vi "bob tilt from parameters.vi"(5 "y0":dbl, 6 "z0":dbl, 7 "x0":dbl, 8 "t":dbl, 9 "phi_dot":dbl, 10 "phi0":dbl, 11 "bob tilt":dbl) -> (2 "derivatives (i,j) = dOut(i) / dParam(j)":dbl[][](array[numeric]), 3 "Out = (x,y,z,tx,ty,BrV)":dbl[](array[numeric]))   [LabVIEW 2017]
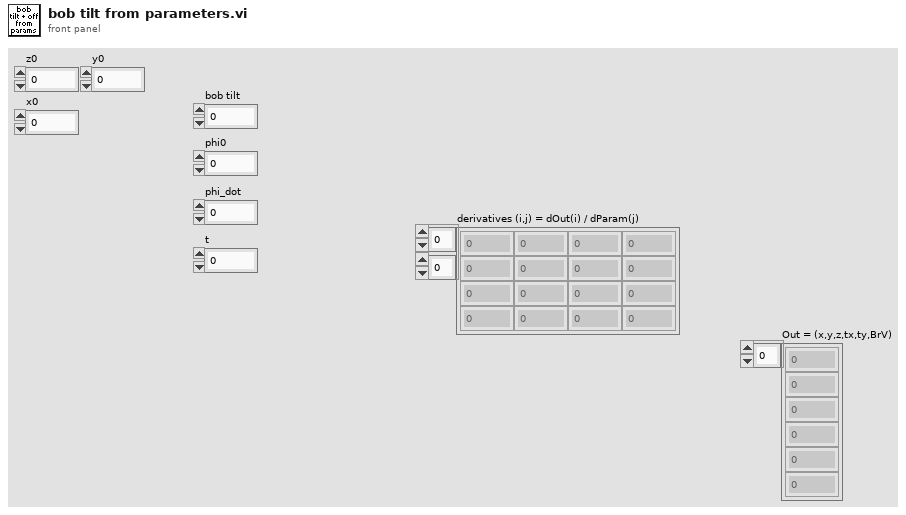
[diagram p1: front panel]
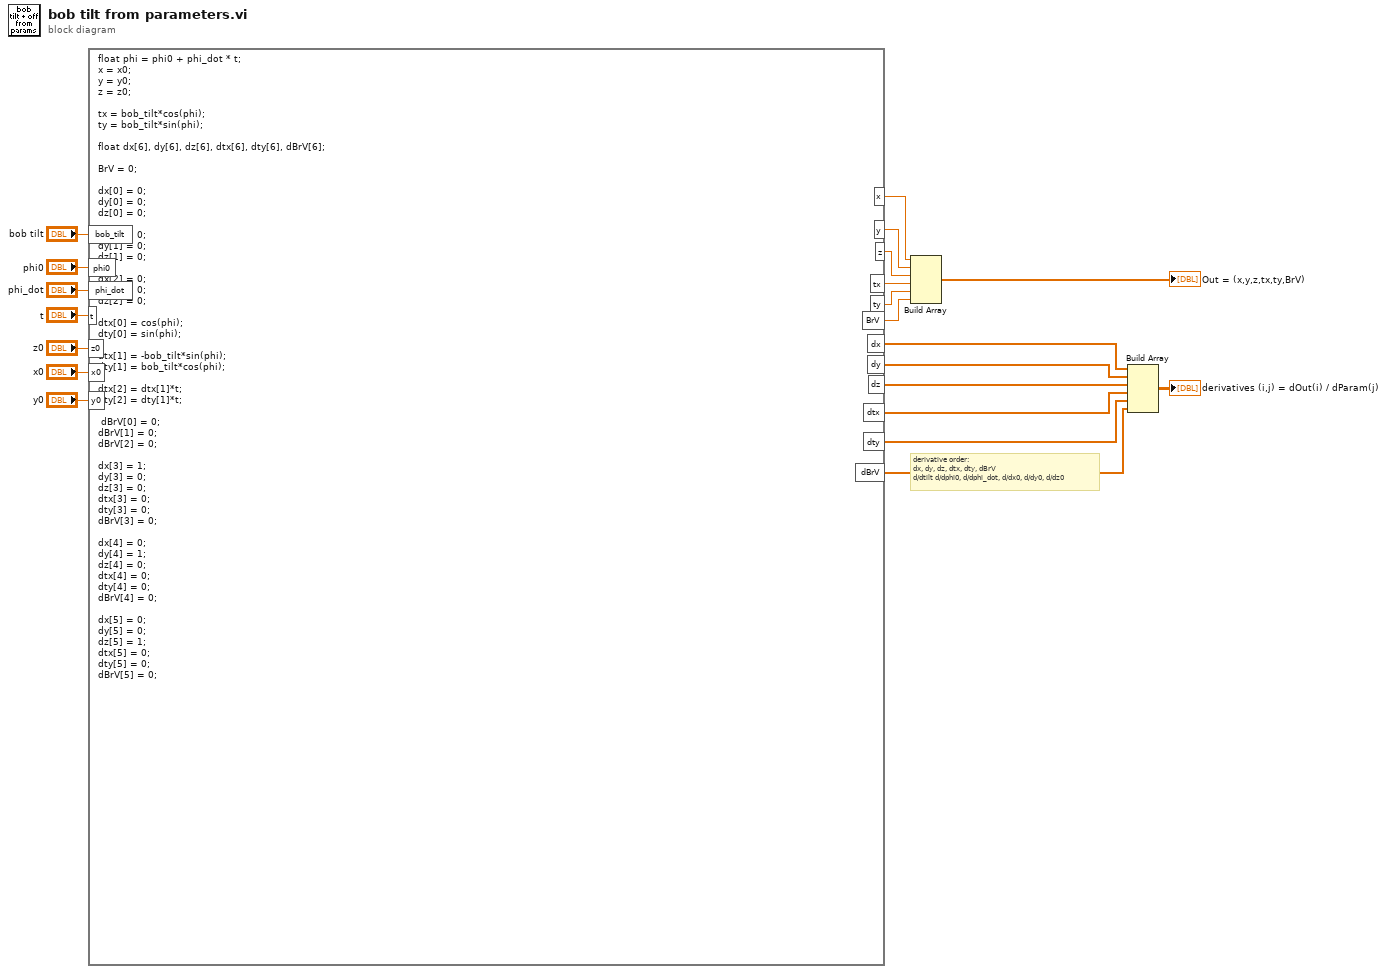
[diagram p0: block diagram]
diagram:
  # "derivative order:\ndx, dy, dz, dtx, dty, dBrV\nd/dtilt d/dphi0, d/dphi_dot, d/dx0, d/dy0, d/dz0"
  n1 = formula code="float phi = phi0 + phi_dot * t;\nx = x0;\ny = y0;\nz = z0;\n\ntx = bob_tilt*cos(phi);\nty = bob_tilt*sin(phi);\n\nfloat dx[6], dy[6], dz[6], dtx[6], dty[6], dBrV[6];\n\nBrV = 0;\n\ndx[0] = 0;\ndy[0] = 0;\ndz[0] = 0;\n\ndx[1] = 0;\ndy[1] = 0;\ndz[1] = 0;\n\ndx[2] = 0;\ndy[2] = 0;\ndz[2] = 0;\n\ndtx[0] = cos(phi);\ndty[0] = sin(phi);\n\ndtx[1] = -bob_tilt*sin(phi);\ndty[1] = bob_tilt*cos(phi);\n\ndtx[2] = dtx[1]*t;\ndty[2] = dty[1]*t;\n\n dBrV[0] = 0;\ndBrV[1] = 0;\ndBrV[2] = 0;\n\ndx[3] = 1;\ndy[3] = 0;\ndz[3] = 0;\ndtx[3] = 0;\ndty[3] = 0;\ndBrV[3] = 0;\n\ndx[4] = 0;\ndy[4] = 1;\ndz[4] = 0;\ndtx[4] = 0;\ndty[4] = 0;\ndBrV[4] = 0;\n\ndx[5] = 0;\ndy[5] = 0;\ndz[5] = 1;\ndtx[5] = 0;\ndty[5] = 0;\ndBrV[5] = 0;"("t"="t", "bob_tilt"="bob tilt", "phi0"="phi0", "phi_dot"="phi_dot", "z0"="z0", "x0"="x0", "y0"="y0") -> ("x"=w12:dbl, "y"=w11:dbl, "z"=w10:dbl, "tx"=w9:dbl, "dx"=w15:dbl[], "dy"=w16:dbl[], "dz"=w17:dbl[], "dtx"=w13:dbl[], "ty"=w7:dbl, "dty"=w6:dbl[], "dBrV"=w5:dbl[], "BrV"=w1:dbl)
  n2 = Build Array(w12, w11, w10, w9, w7, w1) -> (→"Out = (x,y,z,tx,ty,BrV)":dbl[])
  n3 = Build Array(w15, w16, w17, w13, w6, w5) -> (→"derivatives (i,j) = dOut(i) / dParam(j)":dbl[][])
